vi "ChkUpdate.vi"(9 "ChkUpdateCnt":refnum<vi>, 10 "Settings":refnum<vi>) -> (1 "FoundNew":bool, 2 "NewVersion":string)   [LabVIEW 2015]
uses:
  <vilib>/Utility/sysdir.llb/System Directory Type.ctl
  <vilib>/WebDAVClient/Simple Get File.vi
  <vilib>/Utility/config.llb/Write Key (Boolean).vi
  <vilib>/Utility/config.llb/Write Key (String).vi
  <vilib>/Utility/config.llb/Write Key (Double).vi
  <vilib>/WebDAVClient/NI_WebDAV.lvlib
  <vilib>/Utility/config.llb/NI_LVConfig.lvlib
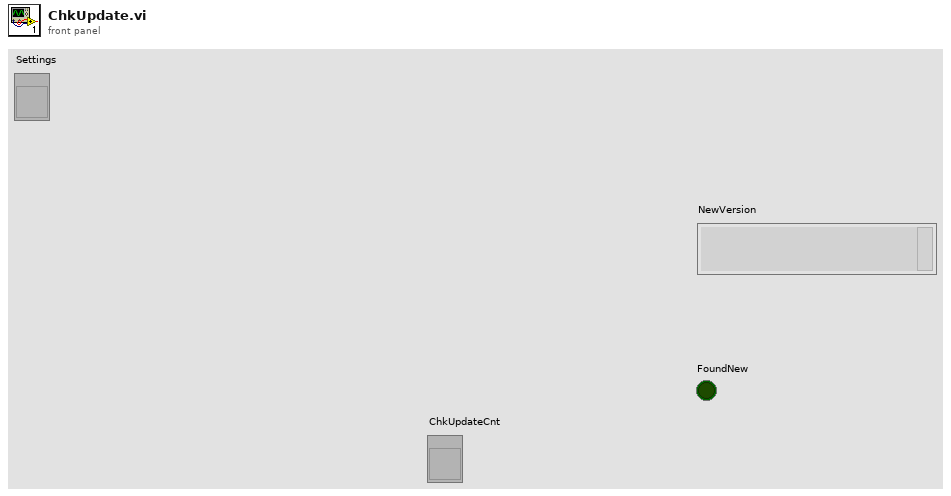
[diagram p1: front panel]
types:
  T1 = typedef "System Directory Type.ctl" = i32
  T2 = typedef "SettingParameters.ctl" = cluster{"LangSet":u32, "TimeFormat":u16, "TimeRerange":bool, "isAutoCurves":bool, "isAutoY":bool, "NeedUpdate":bool, "LastTimChkUpdate":dbl, "NewVersionOnWeb":string, "ChkUpdatePeriod":u32, "LineWidth":u8, "isShowYValue":bool, "isShowXY":bool}
  T3 = typedef "NI_LVConfig.lvlib/Config Data RefNum.ctl" = refnum<k1>
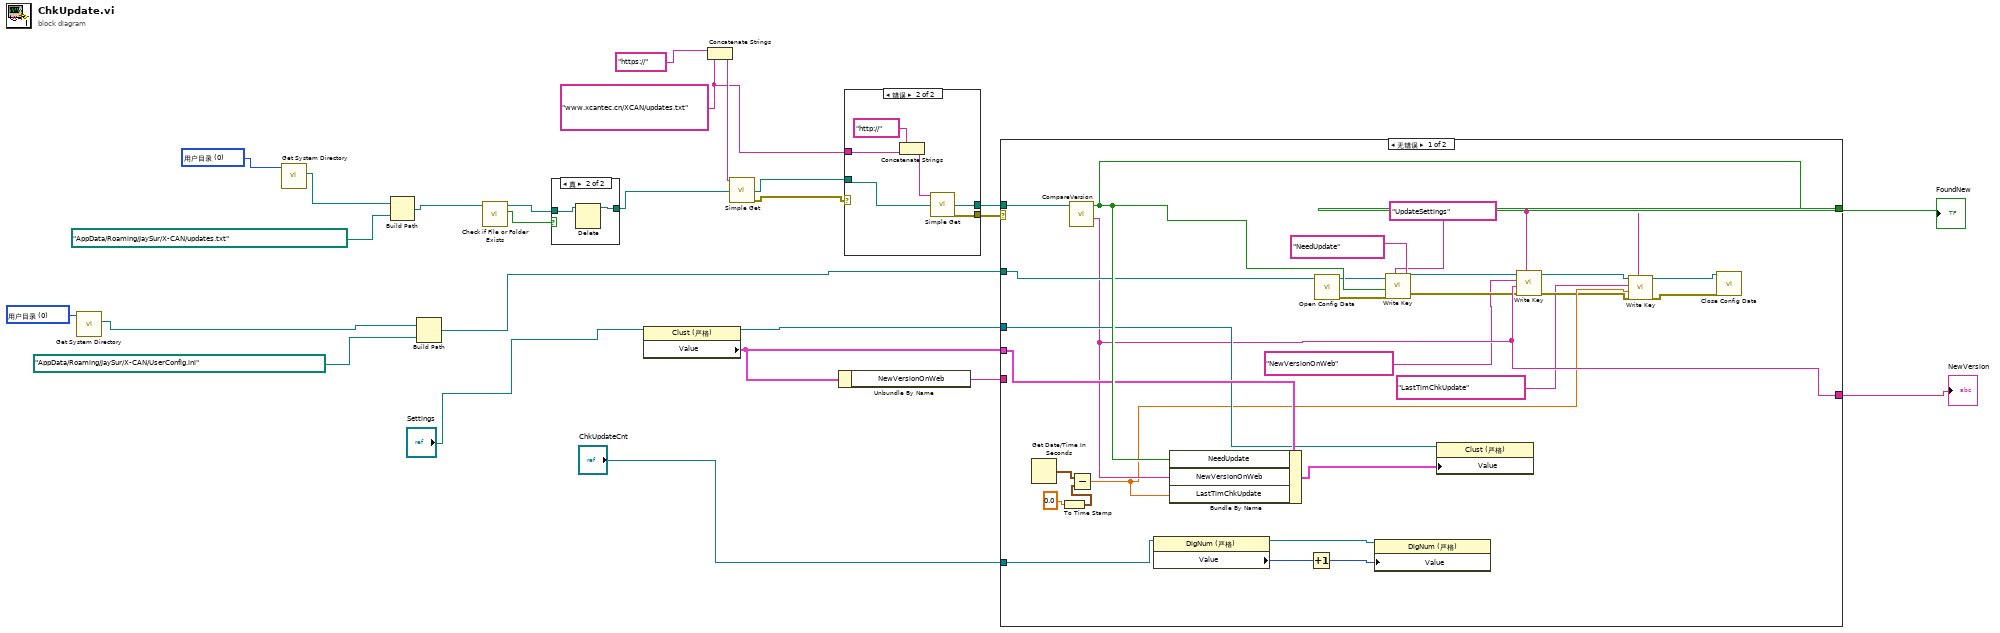
[diagram p0: block diagram]
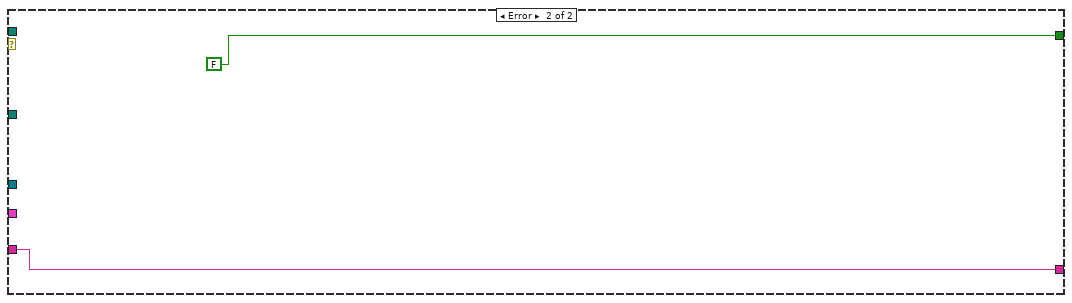
[diagram p3: hidden frame]
diagram:
  w11 = T1 0 items=["用户目录"=0, "用户桌面"=1, "用户文档"=2, "用户应用程序数据"=3, "用户设置"=4, "用户临时目录"=5, "公共文档"=6, "公共应用程序数据"=7, "公共设置"=8, "公共缓存"=13, "系统核心库"=9, "系统安装库"=10, "应用程序文件"=11, "启动盘根目录"=12] ("system directory type")
  w20 = T1 0 items=["用户目录"=0, "用户桌面"=1, "用户文档"=2, "用户应用程序数据"=3, "用户设置"=4, "用户临时目录"=5, "公共文档"=6, "公共应用程序数据"=7, "公共设置"=8, "公共缓存"=13, "系统核心库"=9, "系统安装库"=10, "应用程序文件"=11, "启动盘根目录"=12] ("system directory type")
  w23 = "www.xcantec.cn/XCAN/updates.txt" ("remote file uri")
  n1 = call <vilib>:"Get System Directory.vi"("system directory type"=w11) -> ("system directory"=w12:path)  [unwired: 10 in]
  n2 = call <vilib>:"Get System Directory.vi"("system directory type"=w20) -> ("system directory"=w21:path)  [unwired: 10 in]
  n3 = Build Path(base path=w21, name or relative path=path "AppData/Roaming/JaySur/X-CAN/updates.txt" ("default name")) -> (appended path=w17:path)
  n4 = Build Path(base path=w12, name or relative path=path "AppData/Roaming/JaySur/X-CAN/UserConfig.ini" ("default name")) -> (appended path=w10:path)
  n5 = call <vilib>:"Check if File or Folder Exists.vi"("path"=w17) -> ("file or folder exists?"=w19:bool, "dup path"=w18:path)  [unwired: 8 in, 1 out]
  n6 = case shown="真" w19 {
    tunnel: w18 -> [w26 w28]
    tunnel: [w26 w27] -> w16
    frame False {
    }
    frame True {
      n7 = Delete(path (use dialog)=w28) -> (deleted path=w27:path)  [unwired: 4 in, 2 out]
    }
  }
  n8 = property class="Clust (严格)"(reference="Settings") -> (reference out=w9:refnum<vi>, "Value"=w8:T2)  [unwired: 1 in, 1 out]
  n9 = Concatenate Strings("https://", w23) -> (w24:string)
  n10 = call-poly <vilib>:"Simple Get.vi"("remote file uri"=w24, "local file path"=w16) -> ("local file path out"=w15:path, "error out"=w2:errorcluster)  [unwired: 12 in]
  n11 = Unbundle By Name(w8) -> ("NewVersionOnWeb"=w3:string)
  n12 = case shown="错误" w2 {
    selector: w2 -> [w29 _]
    tunnel: w23 -> [_ w36]
    tunnel: w15 -> [w30 w35]
    tunnel: [w29 w34] -> w5
    tunnel: [w30 w31] -> w4
    frame No Error {
    }
    frame Error {
      n13 = Concatenate Strings("http://", w36) -> (w32:string)
      n14 = call-poly <vilib>:"Simple Get.vi"("remote file uri"=w32, "local file path"=w35) -> ("local file path out"=w31:path, "error out"=w34:errorcluster)  [unwired: 12 in]
    }
  }
  n15 = case shown="无错误" w5 {
    tunnel: w4 -> [w63 _]
    tunnel: [w61 FALSE] -> w14
    tunnel: w9 -> [w58 _]
    tunnel: w10 -> [w60 _]
    tunnel: w8 -> [w59 _]
    tunnel: [w57 w64] -> w7
    tunnel: w3 -> [_ w64]
    tunnel: "ChkUpdateCnt" -> [w40 _]
    frame No Error {
      w44 = "UpdateSettings" ("section")
      n16 = Get Date/Time In Seconds() -> (seconds since 1Jan1904=w56:timestamp)
      n17 = To Time Stamp(1:0.0) -> (0:w54:timestamp)
      n18 = call "CompareVersion.vi"("local file path out"=w63) -> ("NewVersion"=w57:string, "FoundNew"=w61:bool)  [unwired: 9 in]
      n19 = Subtract(x=w56, y=w54) -> (x-y=w53:dbl)
      n20 = property class="DigNum (严格)"(reference=w40) -> (reference out=w37:refnum<vi>, "Value"=w39:i32)  [unwired: 1 in, 1 out]
      n21 = Bundle By Name(cluster=w59, "NeedUpdate"=w61, "NewVersionOnWeb"=w57, "LastTimChkUpdate"=w53) -> (w62:T2)
      n22 = Increment(x=w39) -> (x+1=w38:i32)
      n23 = call <vilib>:"Open Config Data.vi"("configuration file path"=w60) -> ("error out"=w49:errorcluster, "refnum"=w50:T3)  [unwired: 8 in, 1 out]
      n24 = property class="DigNum (严格)"(reference=w37, "Value"=w38) -> ()  [unwired: 1 in, 2 out]
      n25 = call-poly <vilib>:"Write Key.vi"("section"=w44, "error in (no error)"=w49, "value"=w61, "key"="NeedUpdate", "refnum"=w50) -> ("error out"=w51:errorcluster, "refnum out"=w52:T3)  [unwired: 4 in, 1 out]
      n26 = property class="Clust (严格)"(reference=w58, "Value"=w62) -> ()  [unwired: 1 in, 2 out]
      n27 = call-poly <vilib>:"Write Key.vi"("section"=w44, "error in (no error)"=w51, "value"=w57, "key"="NewVersionOnWeb", "refnum"=w52) -> ("error out"=w45:errorcluster, "refnum out"=w46:T3)  [unwired: 4 in, 1 out]
      n28 = call-poly <vilib>:"Write Key.vi"("section"=w44, "error in (no error)"=w45, "value"=w53, "key"="LastTimChkUpdate", "refnum"=w46) -> ("error out"=w41:errorcluster, "refnum out"=w42:T3)  [unwired: 4 in, 1 out]
      n29 = call <vilib>:"Close Config Data.vi"("error in (no error)"=w41, "refnum"=w42) -> ()  [unwired: 8 in, 2 out]
    }
    frame Error {
    }
  }
  "FoundNew" <- w14
  "NewVersion" <- w7
